vi "GetImageData.vi"() -> (0 "ImageData":u16[](array[numeric]))   [LabVIEW 2014]
panel:
  out "NumPixels":i32
  in  "AmpNumber":dbl
  in  "LastPixel":i32=-1
  in  "FirstPixel":i32
  in  "Close":bool
  in  "GetData":bool
  out "Error":bool
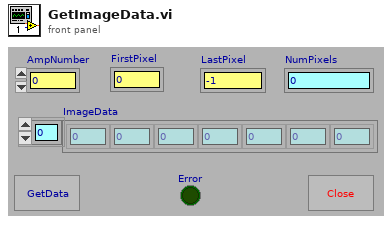
[diagram p1: front panel]
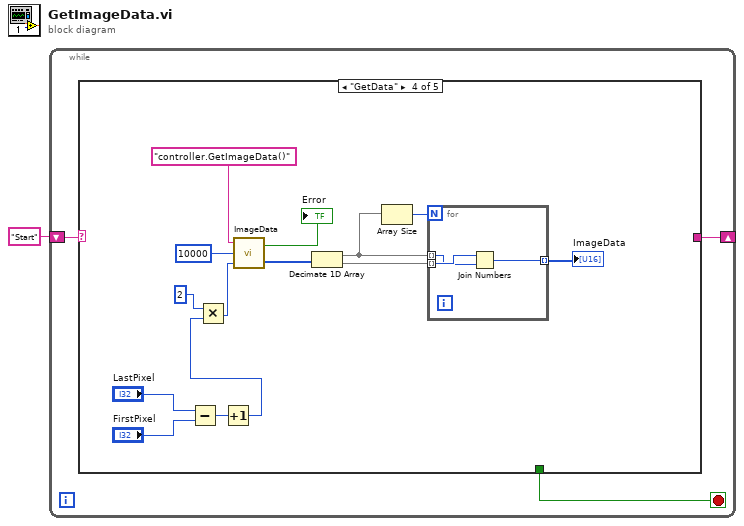
[diagram p0: block diagram]
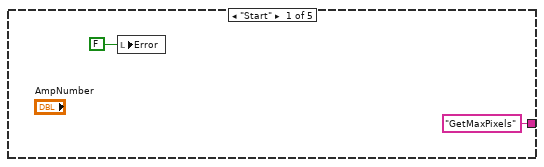
[diagram p2: hidden frame]
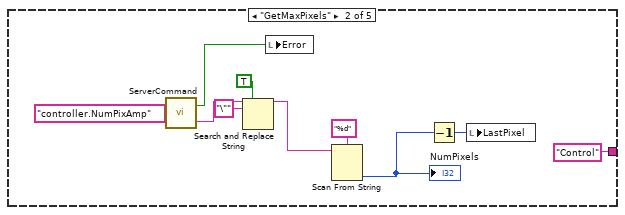
[diagram p3: hidden frame]
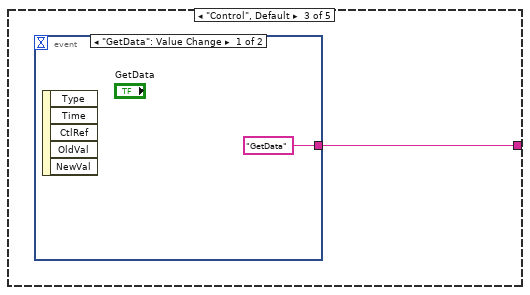
[diagram p4: hidden frame]
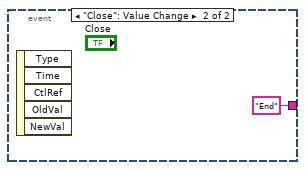
[diagram p5: hidden frame]
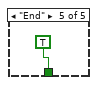
[diagram p6: hidden frame]
diagram:
  n1 = while {
    shift-right: [w3] -> _
    shift-left: "Start" -> [w4]
    stop <- w2 stop-if-true
    n2 = case shown="\"GetData\"" w4 {
      tunnel: ["GetMaxPixels" "Control" w17 _ _] -> w3
      tunnel: [_ _ _ _ TRUE] -> w2
      frame "Start" {
        n3 = local write "Error"(FALSE ("Error")) -> ()
      }
      frame "GetMaxPixels" {
        n4 = call "ServerCommand.vi"("Command"="controller.NumPixAmp") -> ("Error"=w7:bool, "Reply"=w12:string)
        n5 = Search and Replace String(replace all?=TRUE ("replace all? (F)"), input string=w12, search string="\"") -> (result string=w9:string)  [unwired: 5 in, 3 out]
        n6 = local write "Error"(w7) -> ()
        n7 = Scan From String(format string="%d", input string=w9) -> (output 1=w13:i32)  [unwired: 3 in, 3 out]
        "NumPixels" <- w13
        n8 = Decrement(x=w13) -> (x-1=w8:i32)
        n9 = local write "LastPixel"(w8) -> ()
      }
      frame "Control", Default {
        n10 = event shown="[0] \"GetData\": Value Change" {
          selector: _ -> [_ _]
          dyn-events: _ -> [_ _]
          timeout: _ -> [_ _]
          tunnel: ["GetData" "End"] -> w17
          event "GetData": Value Change {
            n11 = event-data() -> ()  [unwired: 1 in, 5 out]
          }
          event "Close": Value Change {
            n12 = event-data() -> ()  [unwired: 1 in, 5 out]
          }
        }
      }
      frame "GetData" {
        n13 = Subtract(x="LastPixel", y="FirstPixel") -> (x-y=w22:i32)
        n14 = Increment(x=w22) -> (x+1=w21:i32)
        n15 = Multiply(x=2, y=w21) -> (x*y=w25:i32)
        n16 = call "ImageData.vi"("bytes to read"=w25, "timeout ms"=10000, "command"="controller.GetImageData()") -> ("unsigned byte array"=w30:u8[], "Error"=→"Error":bool)
        n17 = Decimate 1D Array(w30) -> (w27:u8[], w29:u8[])
        n18 = Array Size(array=w27) -> (size(s)=w28:i32)
        n19 = for {
          N: w28 -> [_]
          tunnel: w29 -> [w35] mode=indexing
          tunnel: w27 -> [w34] mode=indexing
          tunnel: [w36] -> w20 mode=indexing
          n20 = Join Numbers(hi=w35, lo=w34) -> ((hi.lo)=w36:u16)
        }
        "ImageData" <- w20
      }
      frame "End" {
      }
    }
  }
